vi "init_memtest_1channel.vi"(6 "memtest":T1={"Samples to Read"=1000, "Rate (Hz)"=20000.0, "Amplitude (mV/pA)"=10.0, "Offset (mV/pA)"=-60.0, "Frequency (Hz)"=-60.0, "duty cycle (%)"=50.0, "phase"=0.0} {"phase" format="%.2p"; "duty cycle (%)" format="%0.2f"}, 8 "AO error in":errorcluster, 9 "AO physical channels":tag="cDAQ1Mod3/ao14", 10 "AI error in":errorcluster, 11 "AI Physical Channels":tag="cDAQ1Mod1/ai0") -> (0 "AO error out":errorcluster, 1 "AO task out":refnum<k21>, 2 "AI error out":errorcluster, 3 "AI task out":refnum<k21>, 4 "view memtest":waveform(dbl)(graph))   [LabVIEW 2019]
uses:
  controls/memtest_def.ctl
  <vilib>/DAQmx/write.llb/DAQmx Write (Analog Wfm 1Chan NSamp).vi
  <vilib>/DAQmx/create/channels.llb/DAQmx Create Channel (AI-Voltage-Basic).vi
  <vilib>/DAQmx/create/channels.llb/DAQmx Create Channel (AO-Voltage-Basic).vi
  <vilib>/DAQmx/configure/timing.llb/DAQmx Timing (Sample Clock).vi
  <vilib>/DAQmx/configure/trigger.llb/DAQmx Start Trigger (Digital Edge).vi
  <vilib>/DAQmx/miscellaneous.llb/DAQmx Fill In Error Info.vi
panel:
  in  "which clamp":enum16{"VClamp", "IClamp"}(ring)
  # "init memtest"
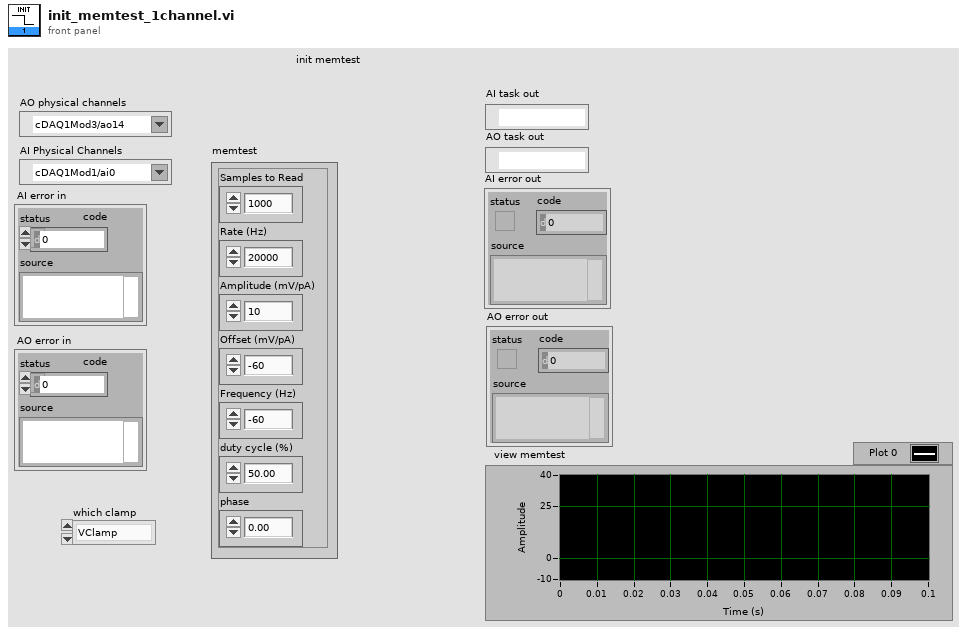
[diagram p1: front panel]
types:
  T1 = typedef "memtest_def.ctl" = cluster{"Samples to Read":i32, "Rate (Hz)":dbl, "Amplitude (mV/pA)":dbl, "Offset (mV/pA)":dbl, "Frequency (Hz)":dbl, "duty cycle (%)":dbl, "phase":dbl}
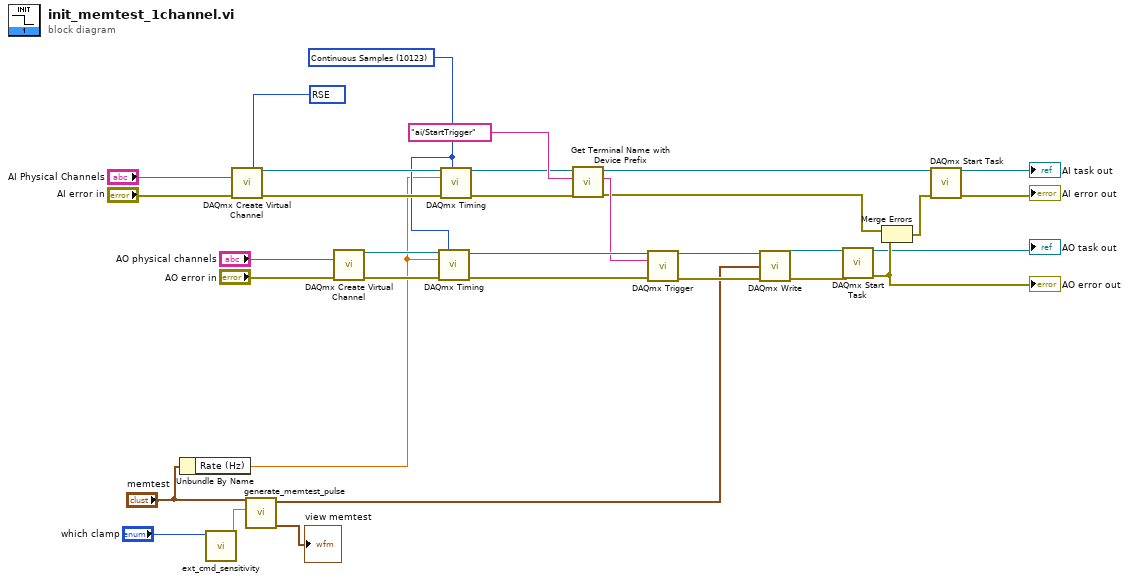
[diagram p0: block diagram]
diagram:
  w30 = 10083 items=["default"=-1, "RSE"=10083, "NRSE"=10078, "Differential"=10106, "Pseudodifferential"=12529] ("input terminal configuration")
  w21 = 10123 items=["Finite Samples"=10178, "Continuous Samples"=10123] ("sample mode")
  n1 = Unbundle By Name("memtest") -> ("Rate (Hz)"=w5:dbl)
  n2 = call "ext_cmd_sensitivity.vi"("which clamp"="which clamp") -> ("division factor"=w3:dbl)  [unwired: 10 in]
  n3 = call-poly <vilib>:"DAQmx Create Virtual Channel.vi"("input terminal configuration"=w30, "physical channels"="AI Physical Channels", "error in"="AI error in") -> ("task out"=w32:refnum<k21>, "error out"=w33:errorcluster)  [unwired: 11 in]
  n4 = call "generate_memtest_pulse.vi"("external cmd sensitivity"=w3, "memtest"="memtest") -> ("view memtest"=→"view memtest":waveform(dbl), "command memtest"=w2:waveform(dbl))  [unwired: 8 in]
  n5 = call-poly <vilib>:"DAQmx Create Virtual Channel.vi"("physical channels"="AO physical channels", "error in"="AO error in") -> ("task out"=w23:refnum<k21>, "error out"=w22:errorcluster)  [unwired: 12 in]
  n6 = call-poly <vilib>:"DAQmx Timing.vi"("task/channels in"=w23, "sample mode"=w21, "rate"=w5, "error in"=w22) -> ("task out"=w19:refnum<k21>, "error out"=w20:errorcluster)  [unwired: 10 in]
  n7 = call-poly <vilib>:"DAQmx Timing.vi"("task/channels in"=w32, "sample mode"=w21, "rate"=w5, "error in"=w33) -> ("task out"=w27:refnum<k21>, "error out"=w26:errorcluster)  [unwired: 10 in]
  n8 = call "Get Terminal Name with Device Prefix.vi"("error in (no error)"=w26, "Local Terminal Name"="ai/StartTrigger" ("terminal"), "task/channels in"=w27) -> ("error out"=w15:errorcluster, "Terminal Name with Device Prefix"=w18:tag, "task out"=w10:refnum<k21>)  [unwired: 6 in]
  n9 = call-poly <vilib>:"DAQmx Trigger.vi"("task/channels in"=w19, "source"=w18, "error in"=w20) -> ("task out"=w17:refnum<k21>, "error out"=w16:errorcluster)  [unwired: 11 in]
  n10 = call-poly <vilib>:"DAQmx Write.vi"("task/channels in"=w17, "data"=w2, "error in"=w16) -> ("task out"=w12:refnum<k21>, "error out"=w11:errorcluster)  [unwired: 10 in, 1 out]
  n11 = call <vilib>:"DAQmx Start Task.vi"("task/channels in"=w12, "error in"=w11) -> ("task out"=→"AO task out":refnum<k21>, "error out"=w13:errorcluster)  [unwired: 12 in]
  "AO error out" <- w13
  n12 = Merge Errors(w15, w13) -> (w14:errorcluster)
  n13 = call <vilib>:"DAQmx Start Task.vi"("task/channels in"=w10, "error in"=w14) -> ("task out"=→"AI task out":refnum<k21>, "error out"=→"AI error out":errorcluster)  [unwired: 12 in]
